vi "GetGtagProperties.vi"(1 "parameters":string) -> (0 "Parameters":cluster{"key":string, "value":string}[](array[cluster]))   [LabVIEW 2012]
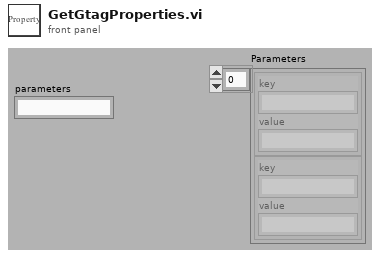
[diagram p1: front panel]
types:
  T1 = cluster{"trimmed string":string, "parameters":string}
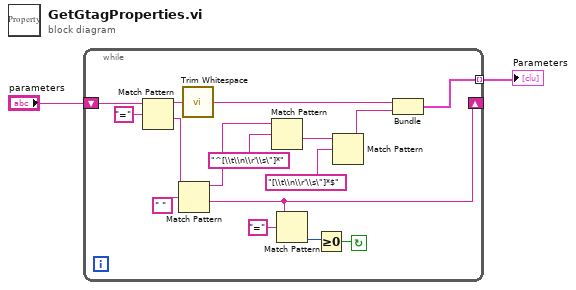
[diagram p0: block diagram]
diagram:
  n1 = while {
    shift-right: [w3] -> _
    shift-left: "parameters" -> [w18]
    tunnel: [w7] -> w2 mode=indexing
    stop <- w4 continue-if-true
    n2 = Match Pattern(string=w18, regular expression="=") -> (before substring=w14:string, after substring=w16:string)  [unwired: 1 in, 2 out]
    n3 = Match Pattern(string=w16, regular expression=" ") -> (before substring=w9:string, after substring=w3:string)  [unwired: 1 in, 2 out]
    n4 = call <vilib>:"Trim Whitespace.vi"("string"=w14) -> ("trimmed string"=w8:string)  [unwired: 1 in]
    n5 = Match Pattern(string=w9, regular expression="^[\\t\\n\\r'\\s\"]*") -> (after substring=w11:string)  [unwired: 1 in, 3 out]
    n6 = Match Pattern(string=w3, regular expression="=") -> (offset past match=w5:i32)  [unwired: 1 in, 3 out]
    n7 = Greater Or Equal To 0?(x=w5) -> (x >= 0?=w4:bool)
    n8 = Match Pattern(string=w11, regular expression="[\\t\\n\\r'\\s\"]*$") -> (before substring=w10:string)  [unwired: 1 in, 3 out]
    n9 = Bundle("trimmed string"=w8, "parameters"=w10) -> (w7:T1)  [unwired: 1 in]
  }
  "Parameters" <- w2
